vi "Digital Parse Configuration Parameters.vi"(10 "Digital Configuration Parameters":T1) -> (1 "name to assign":string, 2 "lines":string, 4 "Active Low":bool)   [LabVIEW 2021]
uses:
  Digital Configuration Parameters.ctl
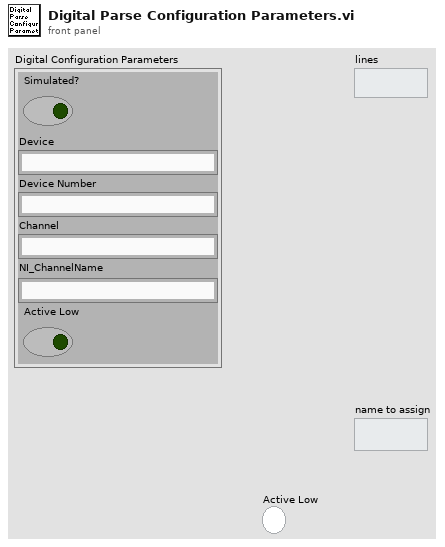
[diagram p1: front panel]
types:
  T1 = typedef "Digital Configuration Parameters.ctl" = cluster{"Simulated?":bool, "Device":string, "Device Number":string, "Channel":string, "NI_ChannelName":string, "Active Low":bool}
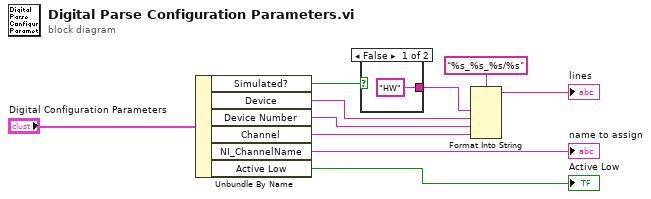
[diagram p0: block diagram]
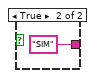
[diagram p2: hidden frame]
diagram:
  n1 = Unbundle By Name("Digital Configuration Parameters") -> ("Simulated?"=w2:bool, "Device"=w7:string, "Device Number"=w5:string, "Channel"=w6:string, "NI_ChannelName"=→"name to assign":string, "Active Low"=→"Active Low":bool)
  n2 = case shown="False" w2 {
    tunnel: ["HW" ("format string") "SIM" ("format string")] -> w1
    frame False {
    }
    frame True {
    }
  }
  n3 = Format Into String(format string="%s_%s_%s/%s", w1, w7, w5, w6) -> (resulting string=→"lines":string)  [unwired: 2 in, 1 out]
